vi "set_task.vi"(8 "error in (no error)":errorcluster, 9 "counter task":refnum<k21>, 10 "output task":refnum<k21>, 11 "DAQmxWriteSignals in":refnum<class "SignalWriterDL090202DAQmx.lvclass">) -> (0 "error out":errorcluster, 3 "DAQmxWriteSignals out":refnum<class "SignalWriterDL090202DAQmx.lvclass">)   [LabVIEW 2010, in "SignalWriterDL090202DAQmx.lvclass"]
uses:
  SignalWriterDL090202DAQmx.lvclass
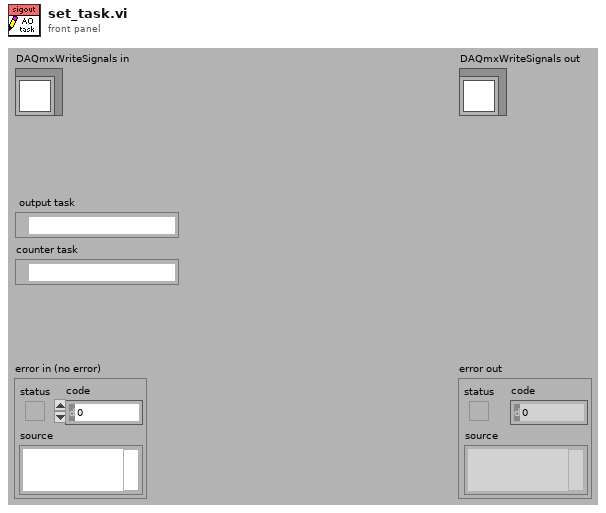
[diagram p1: front panel]
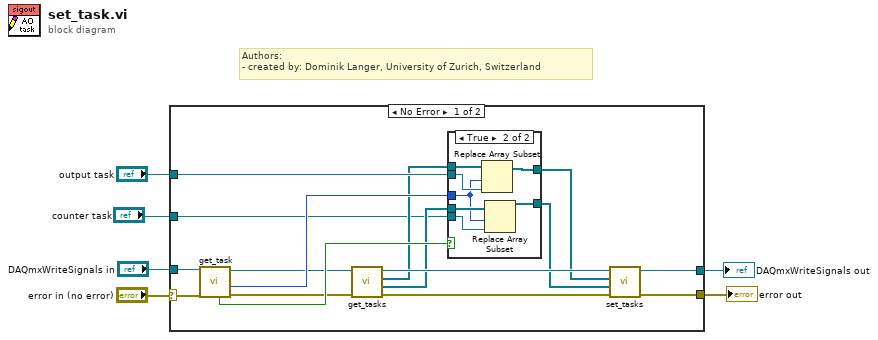
[diagram p0: block diagram]
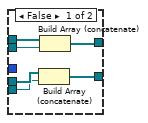
[diagram p2: hidden frame]
diagram:
  # "Authors: \n- created by: Dominik Langer, University of Zurich, Switzerland"
  n1 = case shown="No Error" "error in (no error)" {
    selector: "error in (no error)" -> [w22 w37]
    tunnel: [w16 w37] -> w5
    tunnel: [w12 w36] -> w3
    tunnel: "DAQmxWriteSignals in" -> [w21 w36]
    tunnel: "output task" -> [w19 _]
    tunnel: "counter task" -> [w8 _]
    frame No Error {
      n2 = call-dynamic "get_task.vi"("error in (no error)"=w22, "DAQmxWriteSignals in"=w21) -> ("error out"=w17:errorcluster, "index"=w20:i32, "DAQmxWriteSignals out"=w14:refnum<class "SignalWriterDL090202DAQmx.lvclass">, "found?"=w18:bool)  [unwired: 1 in, 5 out]
      n3 = call-dynamic "get_tasks.vi"("error in (no error)"=w17, "DAQmxWriteSignals in"=w14) -> ("error out"=w15:errorcluster, "counter tasks"=w9:refnum<k21>[], "output tasks"=w10:refnum<k21>[], "DAQmxWriteSignals out"=w13:refnum<class "SignalWriterDL090202DAQmx.lvclass">)  [unwired: 6 out]
      n4 = case shown="True" w18 {
        tunnel: w20 -> [_ w30]
        tunnel: w19 -> [w26 w35]
        tunnel: w10 -> [w28 w34]
        tunnel: [w27 w33] -> w11
        tunnel: w9 -> [w25 w31]
        tunnel: w8 -> [w24 w29]
        tunnel: [w23 w32] -> w7
        frame False {
          n5 = Build Array (concatenate)(w25, w24) -> (w23:refnum<k21>[])
          n6 = Build Array (concatenate)(w28, w26) -> (w27:refnum<k21>[])
        }
        frame True {
          n7 = Replace Array Subset(array=w34, new element=w35, index=w30) -> (w33:refnum<k21>[])
          n8 = Replace Array Subset(array=w31, new element=w29, index=w30) -> (w32:refnum<k21>[])
        }
      }
      n9 = call-dynamic "set_tasks.vi"("error in (no error)"=w15, "counter tasks"=w7, "output tasks"=w11, "DAQmxWriteSignals in"=w13) -> ("error out"=w16:errorcluster, "DAQmxWriteSignals out"=w12:refnum<class "SignalWriterDL090202DAQmx.lvclass">)  [unwired: 6 out]
    }
    frame Error {
    }
  }
  "error out" <- w5
  "DAQmxWriteSignals out" <- w3
